vi "DashBoardGlobals.vi"() -> ()   [LabVIEW 2025]
panel:
  out "Rec Mode":enum32{"Stop", "Record", "Playback"}(radio)
  out "NT Connection":bool
  out "RobotMode":T1(ring)=enum."Auto Disabled"
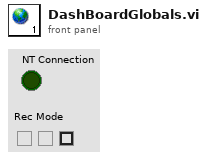
[diagram p1: front panel]
types:
  T1 = enum8{"Tele-Op Disabled", "Tele-Op Enabled", "Auto Disabled", "Auto Enabled", "Test Disabled", "Test Enabled", "Disconnected", "No Code", "E-Stop"}
diagram:
